vi "Swap array elements(CSG).vi"(7 "Swap?":bool=TRUE, 9 "Index2":i32, 10 "Index1":i32, 11 "Input":csg[](array[numeric])) -> (3 "Output":csg[](array[numeric]))   [LabVIEW 2012]
doc: "功能：\n\n交换数组相邻两个元素的值，常见于数组冒泡排序中。\n\nSwap?1布尔输入端子用来选择交换数组的相邻元素，默认为FALSE，不交换。\n\nX[i+1]-->X[i]\n\nX[i]---->X[i+1]\n\ncsxcs_366创建"
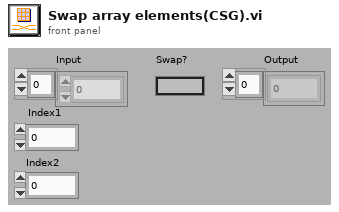
[diagram p1: front panel]
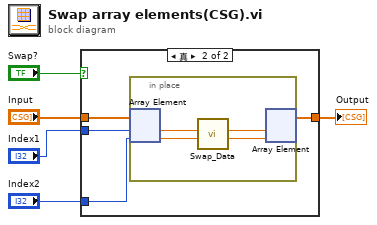
[diagram p0: block diagram]
diagram:
  n1 = case shown="真" "Swap?" {
    tunnel: "Input" -> [w6 w10]
    tunnel: [w6 w9] -> w3
    tunnel: "Index1" -> [_ w8]
    tunnel: "Index2" -> [_ w7]
    frame False {
    }
    frame True {
      n2 = in-place {
        n3 = in-place-array #1(w10, w8, w7) -> (w14:csg, w13:csg)
        n4 = call-poly "Swap_Data.vi"("b"=w13, "a"=w14) -> ("b"=w11:csg, "a"=w12:csg)  [unwired: 5 in]
        n5 = in-place-array #1(w12, w11) -> (w9:csg[])  [unwired: 2 out]
      }
    }
  }
  "Output" <- w3
